vi "Get Available Channels.vi"(8 "error in (no error)":errorcluster, 11 "IO Device in":refnum<class "IO Device.lvclass">) -> (0 "error out":errorcluster, 3 "IO Device out":refnum<class "IO Device.lvclass">)   [LabVIEW 2015, in "IO Device.lvlib" / "IO Device.lvclass"]
uses:
  IO Device.lvclass
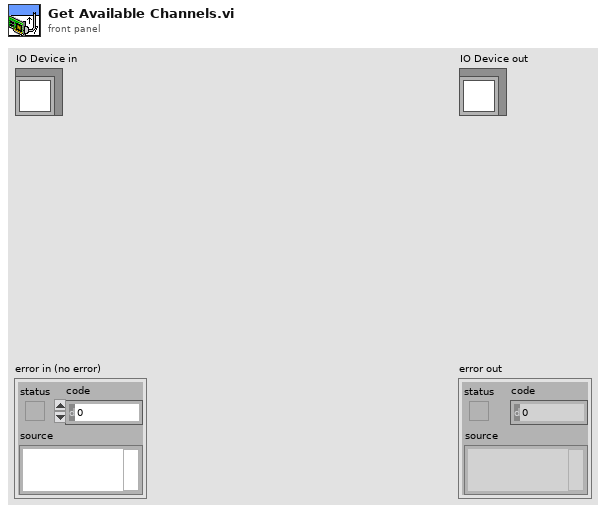
[diagram p1: front panel]
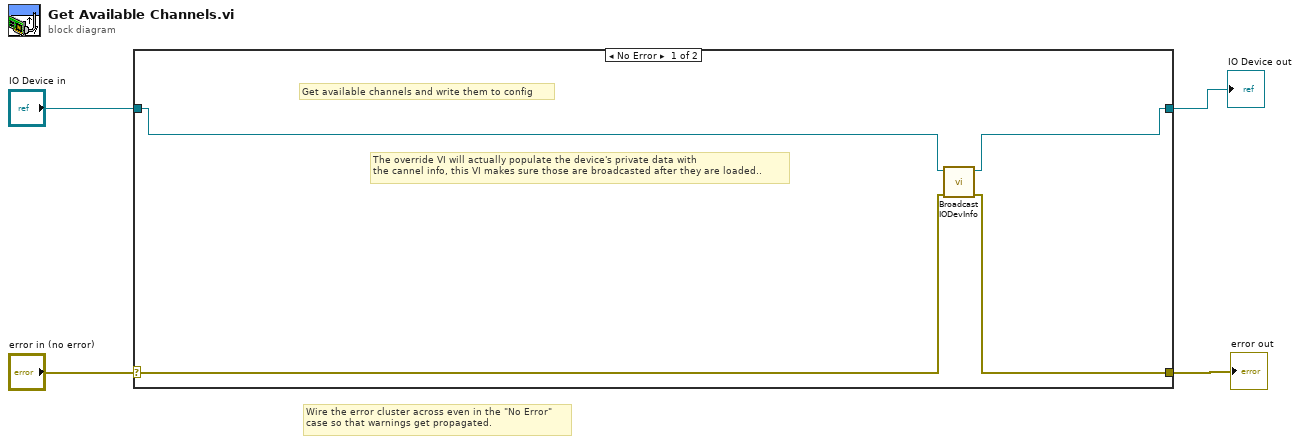
[diagram p0: block diagram]
diagram:
  # "Wire the error cluster across even in the \"No Error\"\ncase so that warnings get propagated."
  n1 = case shown="No Error" "error in (no error)" {
    selector: "error in (no error)" -> [w7 w10]
    tunnel: [w6 w10] -> w3
    tunnel: [w8 w9] -> w1
    tunnel: "IO Device in" -> [w5 w9]
    frame No Error {
      # "The override VI will actually populate the device's private data with \nthe cannel info, this VI makes sure those are broadcasted after they are loaded.."
      # "Get available channels and write them to config"
      n2 = call "Broadcast IODevInfo.vi"("error in (no error)"=w7, "IO Device in"=w5) -> ("error out"=w6:errorcluster, "IO Device out"=w8:refnum<class "IO Device.lvclass">)  [unwired: 8 in]
    }
    frame Error {
    }
  }
  "error out" <- w3
  "IO Device out" <- w1
